vi "build_data_save_paths.vi"(4 "overwrite":bool, 6 "note-blob":string, 7 "meta-file-ext":string=".mat", 8 "error in":errorcluster, 11 "input-file":path) -> (0 "error IO":errorcluster, 1 "output-data-name":string, 2 "output-meta-data-path":path, 3 "output-data-path":path)   [LabVIEW 2017]
uses:
  <vilib>/regexp/Match Regular Expression.xnode
  labview/utils_lib/utils.lvlib
panel:
  out "created path":path
  out "output-meta-data-name":string
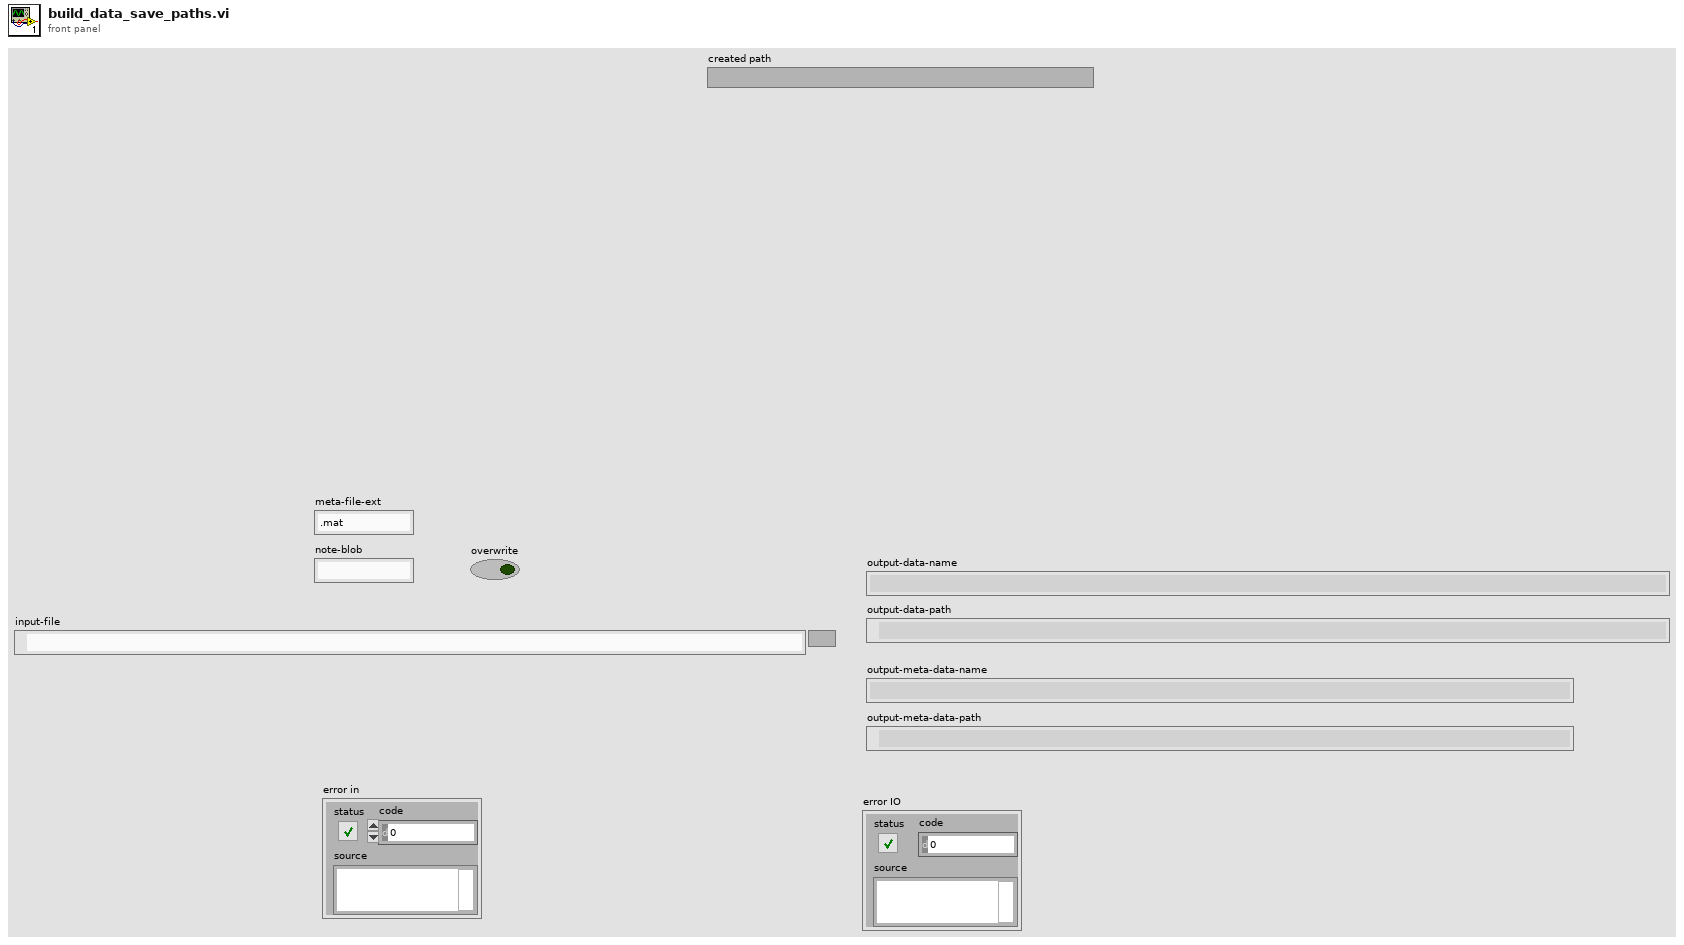
[diagram p1: front panel]
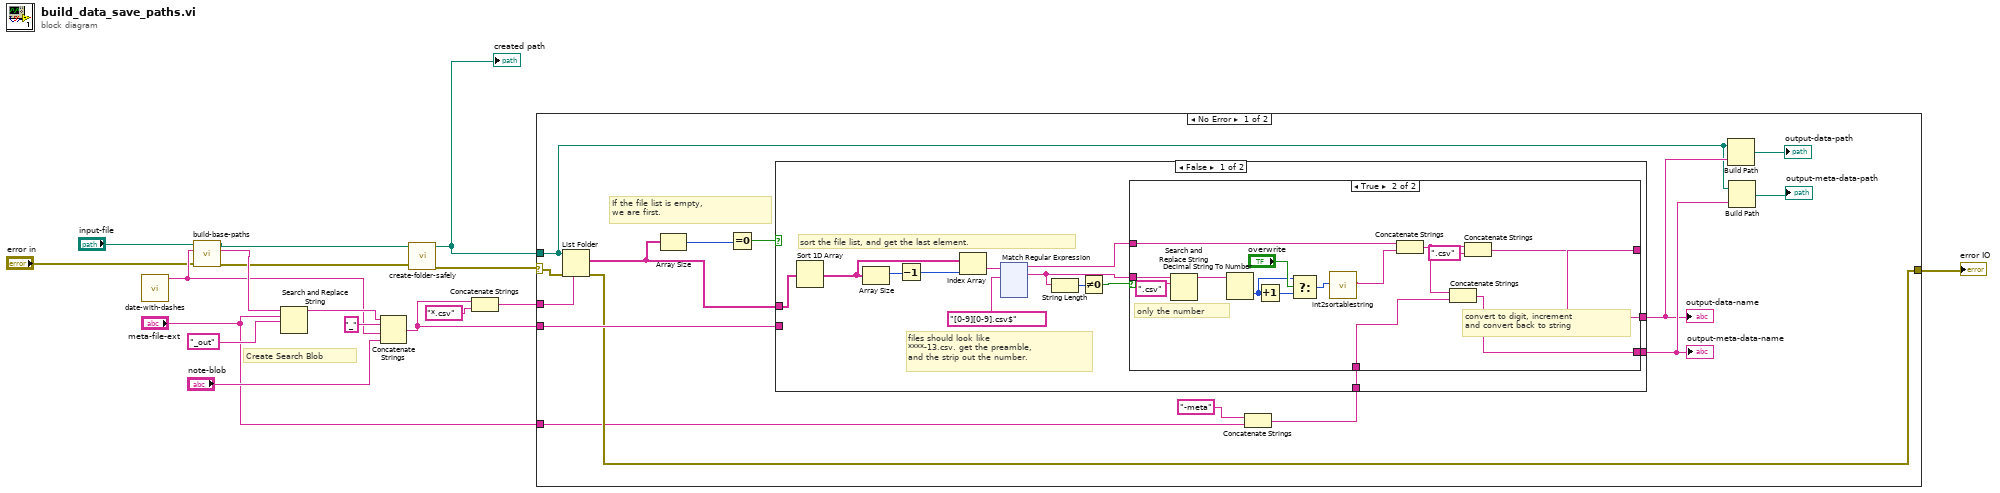
[diagram p0: block diagram]
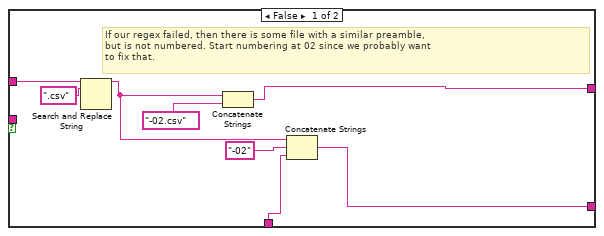
[diagram p2: hidden frame]
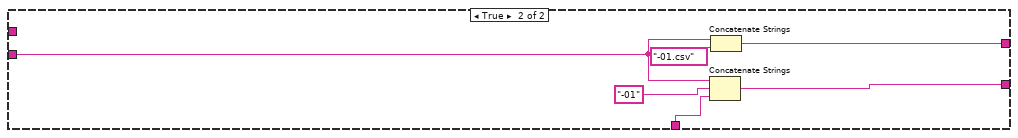
[diagram p3: hidden frame]
diagram:
  # "Create Search Blob"
  n1 = call "date-with-dashes.vi"() -> ("date"=w5:string)  [unwired: 11 in]
  n2 = call "build-base-paths.vi"("error in"="error in", "dest-subfolder"=w5, "input-file"="input-file") -> ("error out"=w3:errorcluster, "input-file-name"=w6:string, "Destination Path"=w7:path)  [unwired: 6 in]
  n3 = Search and Replace String(input string=w6, search string="meta-file-ext", replace string="_out" ("replace string (\"\")")) -> (result string=w17:string)  [unwired: 5 in, 3 out]
  n4 = Concatenate Strings(w17, "_", w5, "note-blob") -> (w12:string)
  n5 = call "create-folder-safely.vi"("error in (no error)"=w3, "folder-path"=w7) -> ("error out"=w10:errorcluster, "created path"=w9:path)  [unwired: 8 in]
  "created path" <- w9
  n6 = Concatenate Strings(w12, "*.csv") -> (w13:string)
  n7 = case shown="No Error" w10 {
    selector: w10 -> [w22 w188]
    tunnel: w13 -> [w30 _]
    tunnel: w12 -> [w29 _]
    tunnel: w9 -> [w23 _]
    tunnel: [w21 w188] -> w2
    tunnel: "meta-file-ext" -> [w18 _]
    frame No Error {
      # "If the file list is empty,\nwe are first."
      n8 = List Folder(path=w23, pattern=w30, error in=w22) -> (filenames=w28:string[], error out=w21:errorcluster)  [unwired: 1 in, 2 out]
      n9 = Array Size(array=w28) -> (size(s)=w32:i32)
      n10 = Equal To 0?(x=w32) -> (x = 0?=w31:bool)
      n11 = Concatenate Strings("-meta" ("string"), w18) -> (w19:string)
      n12 = case shown="False" w31 {
        tunnel: w29 -> [_ w183]
        tunnel: [w39 w185] -> w24
        tunnel: [w38 w184] -> w25
        tunnel: w28 -> [w45 _]
        tunnel: w19 -> [w33 w182]
        frame False {
          # "files should look like\n****-13.csv. get the preamble,\nand the strip out the number."
          # "sort the file list, and get the last element."
          n13 = Sort 1D Array(array=w45) -> (sorted array=w40:string[])
          n14 = Array Size(array=w40) -> (size(s)=w42:i32)
          n15 = Decrement(x=w42) -> (x-1=w41:i32)
          n16 = Index Array(array=w40, index=w41) -> (element=w44:string)
          n17 = xnode "Match Regular Expression"("input string"=w44, "regular expression"="[0-9][0-9].csv$") -> ("before match"=w37:string, "whole match"=w36:string)  [unwired: 4 in, 3 out]
          n18 = String Length(string=w36) -> (length=w35:i32)
          n19 = Not Equal To 0?(x=w35) -> (x != 0?=w34:bool)
          n20 = case shown="True" w34 {
            tunnel: w36 -> [_ w67]
            tunnel: [w51 w62] -> w39
            tunnel: [w52 w61] -> w38
            tunnel: w37 -> [w48 w60]
            tunnel: w33 -> [w46 w54]
            frame False {
              # "If our regex failed, then there is some file with a similar preamble,\nbut is not numbered. Start numbering at 02 since we probably want\nto fix that."
              n21 = Search and Replace String(input string=w48, search string=".csv") -> (result string=w47:string)  [unwired: 6 in, 3 out]
              n22 = Concatenate Strings(w47, "-02.csv" ("string")) -> (w51:string)
              n23 = Concatenate Strings(w47, "-02" ("string"), w46) -> (w52:string)
            }
            frame True {
              # "convert to digit, increment\nand convert back to string"
              # "only the number"
              n24 = Search and Replace String(input string=w67, search string=".csv") -> (result string=w65:string)  [unwired: 6 in, 3 out]
              n25 = Decimal String To Number(string=w65) -> (number=w55:i32)  [unwired: 2 in, 1 out]
              n26 = Increment(x=w55) -> (x+1=w58:i32)
              n27 = Select(t=w55, s="overwrite", f=w58) -> (s? t:f=w57:i32)
              n28 = call "int2sortablestring.vi"("int"=w57) -> ("tens-sortable-string"=w59:string)  [unwired: 10 in]
              n29 = Concatenate Strings(w60, w59) -> (w64:string)
              n30 = Concatenate Strings(w64, w54) -> (w61:string)
              n31 = Concatenate Strings(w64, ".csv" ("string")) -> (w62:string)
            }
          }
        }
        frame True {
          n32 = Concatenate Strings(w183, "-01", w182) -> (w184:string)
          n33 = Concatenate Strings(w183, "-01.csv") -> (w185:string)
        }
      }
      "output-data-name" <- w24
      "output-meta-data-name" <- w25
      n34 = Build Path(base path=w23, name or relative path=w24) -> (appended path=→"output-data-path":path)
      n35 = Build Path(base path=w23, name or relative path=w25) -> (appended path=→"output-meta-data-path":path)
    }
    frame Error {
    }
  }
  "error IO" <- w2
